vi "State Machine.vi"() -> ()   [LabVIEW 2018]
uses:
  <vilib>/Platform/TimedLoop/XDataNode/timing_clust.ctl
  <vilib>/Platform/TimedLoop/XDataNode/nitl_modes.ctl
  <vilib>/Platform/TimedLoop/XDataNode/wakeup.ctl
  <extravilib>/ChannelInstances/Tag-bool/Write With Abort.vi
  <extravilib>/ChannelInstances/Tag-a[.](dbl)/Read With Abort.vi
  <extravilib>/ChannelInstances/Tag-a[.](dbl)/Write With Abort.vi
  <extravilib>/ChannelInstances/Tag-bool/Read With Abort.vi
  <extravilib>/ChannelInstances/Tag-bool/Instantiate.vi
  <extravilib>/ChannelInstances/Tag-a[.](dbl)/Instantiate.vi
  <extravilib>/ChannelInstances/Tag-bool/EndpointRead.vi
  <extravilib>/ChannelInstances/Tag-a[.](dbl)/EndpointRead.vi
  <extravilib>/ChannelInstances/Tag-bool/Endpoint.vi
  <extravilib>/ChannelInstances/Tag-a[.](dbl)/Endpoint.vi
  <vilib>/Platform/TimedLoop/XDataNode/XDataNode.xnode
  <extravilib>/ChannelInstances/Tag-bool.lvlib
  <vilib>/Platform/TimedLoop/XDataNode/XDNodeRunTimeDep.lvlib
  <extravilib>/ChannelInstances/Tag-a[.](dbl).lvlib
panel:
  in  "Reset Button":bool
  out "State":enum16{"Start", "NE", "SE", "NW", "SW", "Reset"}(ring)
  out "error out":errorcluster
  in  "Stop Button":bool
  out "Calibrated":bool=TRUE
  in  "GO?":bool
  out "Stitched Image":T1(plugin-control)
  out "Acquired Image":T1(plugin-control)
  # "Mechatronic Systems Board"
  # "State Machines"
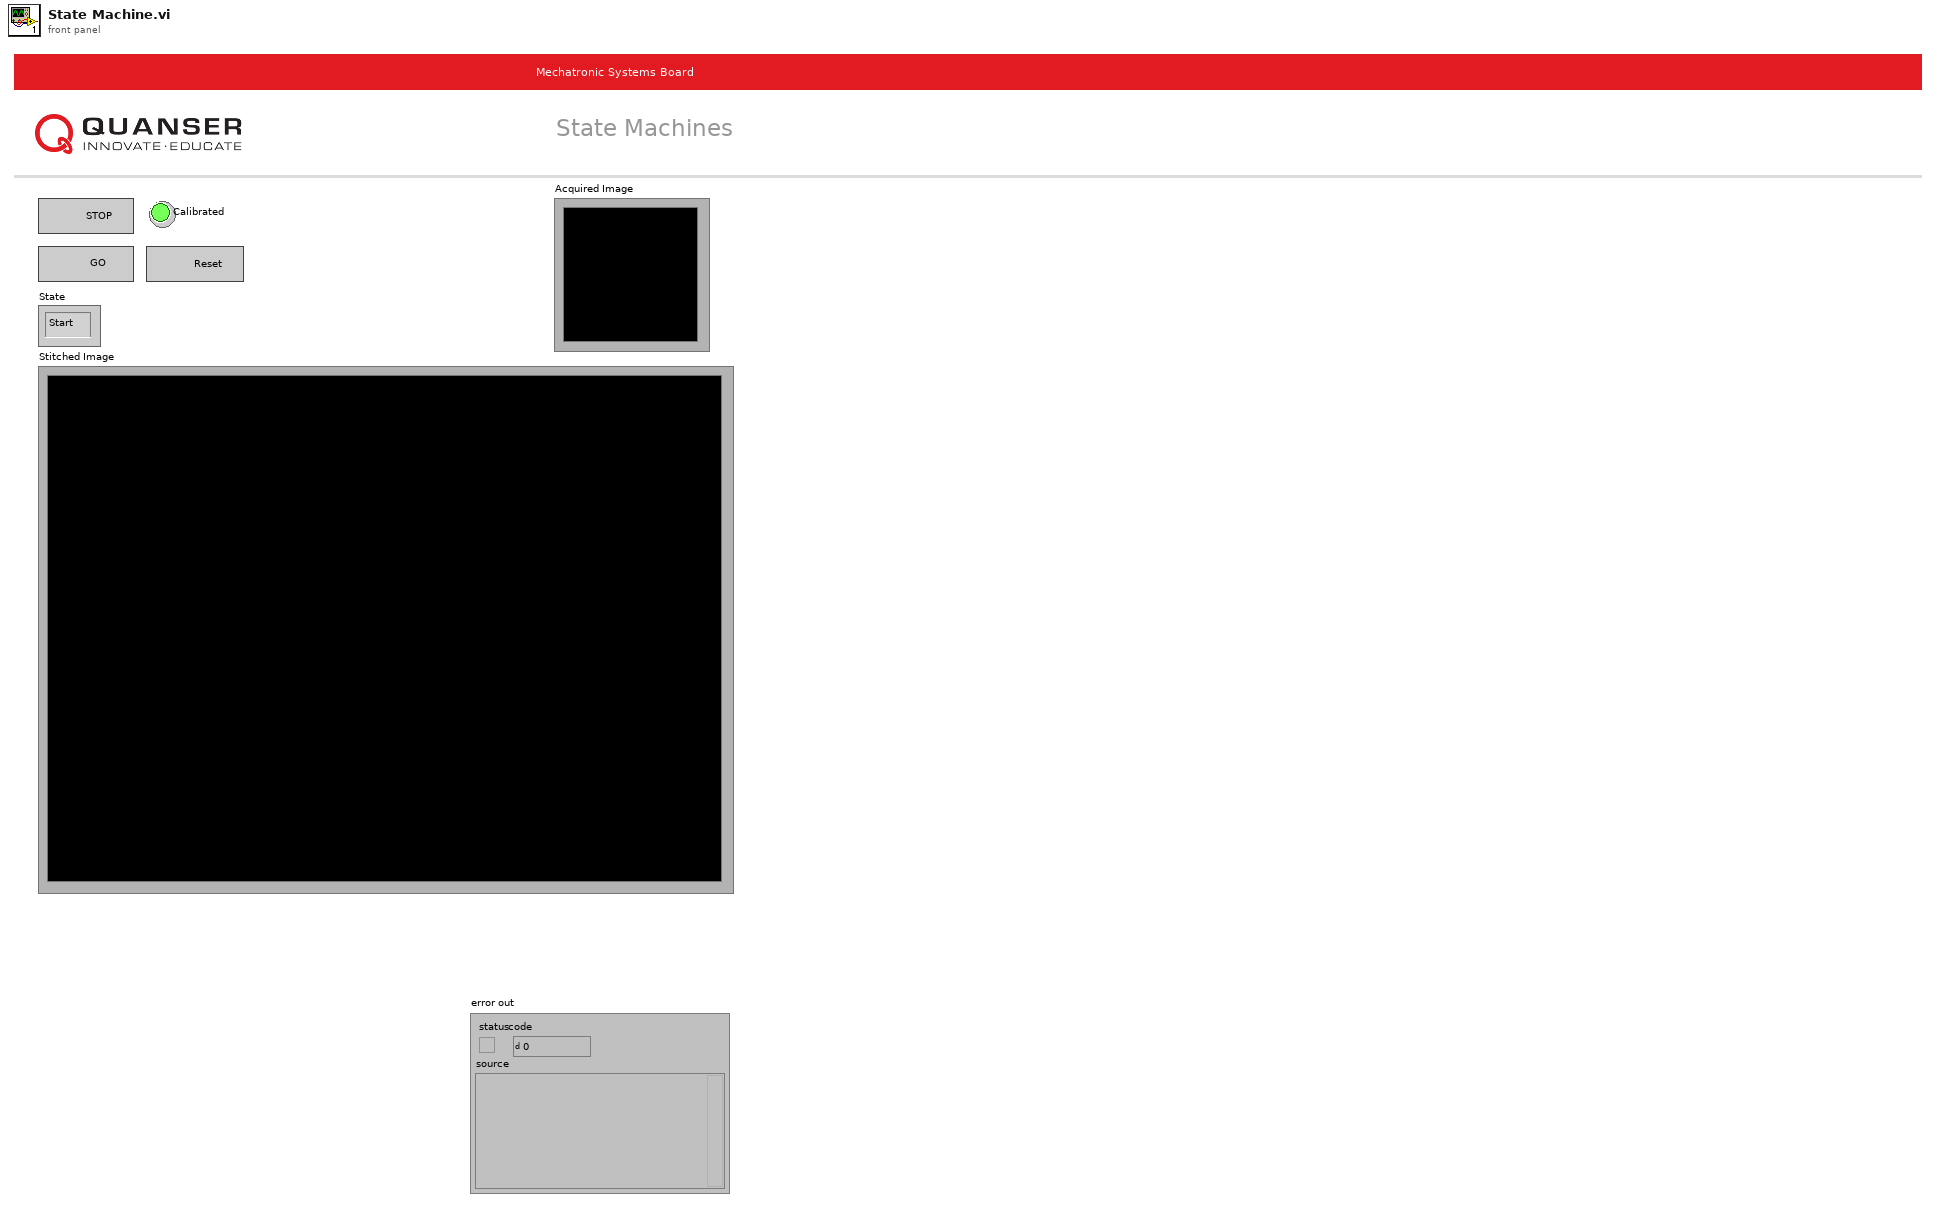
[diagram p1: front panel]
types:
  T1 = typedef "IMAQ Image.ctl" = refnum<image>
  T2 = typedef "QNET MS IO Cluster.ctl" = cluster{"Error":errorcluster, "Encoder Calibration Values":i32[], "Update Calibration":bool, "JPEG Resolutions":u16, "Raw Resolutions":u16, "Image Mode":enum16{"RAW RGB", "RAW Gray Scale", "JPEG"}, "FPGA Ref":refnum<k20>}
  T3 = typedef "XDNodeRunTimeDep.lvlib/timing_clust.ctl" = cluster{"Expected End [f-1]":u64, "Actual End [f-1]":u64, "Finished Late? [f-1]":bool, "Expected End [i-1]":u64, "Actual End [i-1]":u64, "Finished Late? [i-1]":bool, "Expected Start [i]":u64, "Actual Start [i]":u64, "Expected Start [f]":u64, "Actual Start [f]":u64, "Source Name":string, "Structure Name":string, "Period":i64, "Deadline":i64, "Offset":i64, "Start":i64, "Priority":i32, "Timeout":i32, "Mode":T4, "Wakeup Reason":T5, "Error":errorcluster, "Source Type":string, "Secondary Source Type":string, "Global End Time":u64, "Global Start Time":u64, "Frame Duration":u64, "Iteration Duration":u64, "Assigned CPU":i32, "I/O Scan Engine Mode":u32}
  T4 = typedef "XDNodeRunTimeDep.lvlib/nitl_modes.ctl" = enum32{"No Change", "Process missed periods, maintain original phase", "Discard missed periods, maintain original phase", "Process missed periods, ignore original phase", "Discard missed periods, ignore original phase"}
  T5 = typedef "XDNodeRunTimeDep.lvlib/wakeup.ctl" = enum32{"Normal", "Aborted", "Asynchronous wakeup", "Timing source error", "Timed loop error", "Timeout"}
  T6 = typedef "Tag-a[.](dbl).lvlib/))Channel.ctl" = refnum<queue>
  T7 = typedef "Tag-bool.lvlib/))Channel.ctl" = refnum<queue>
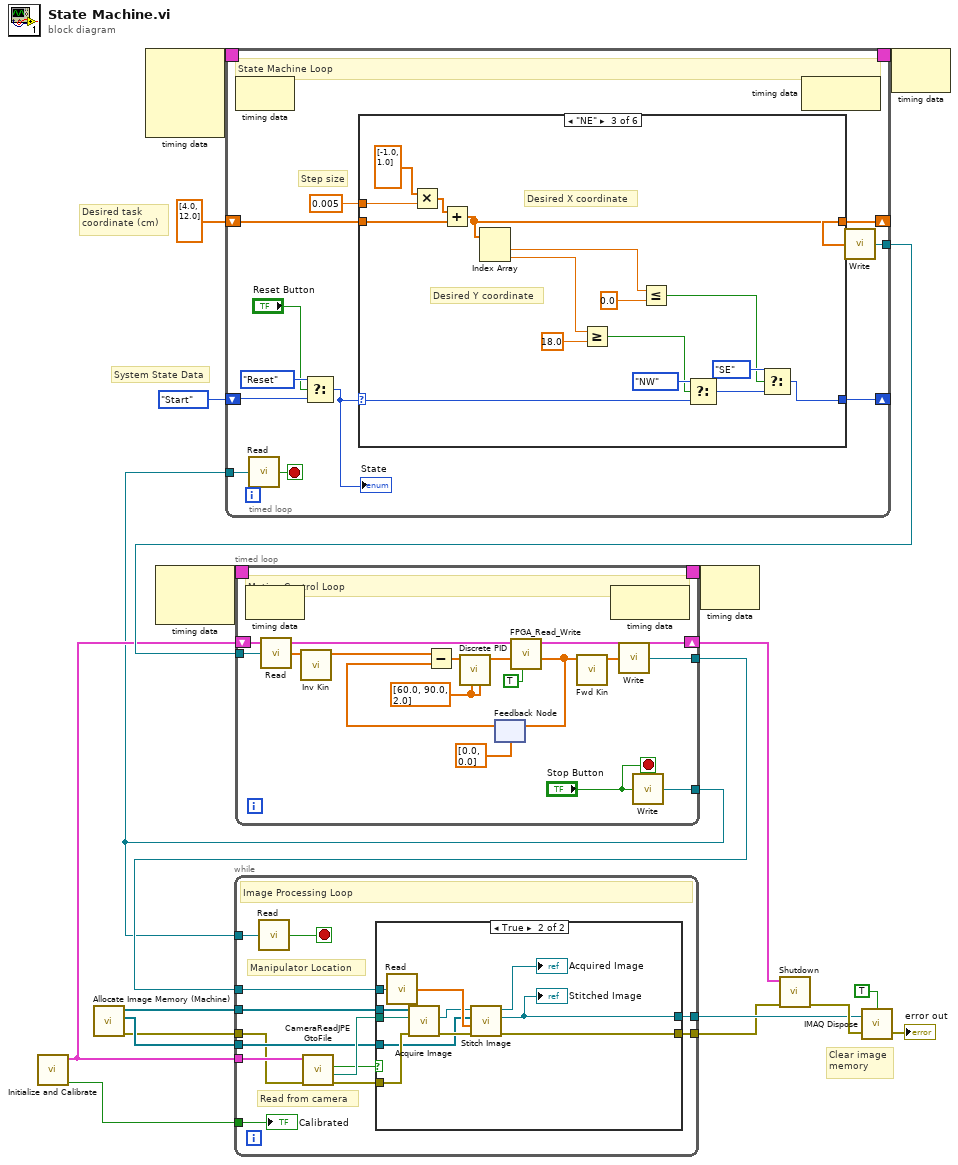
[diagram p0: block diagram]
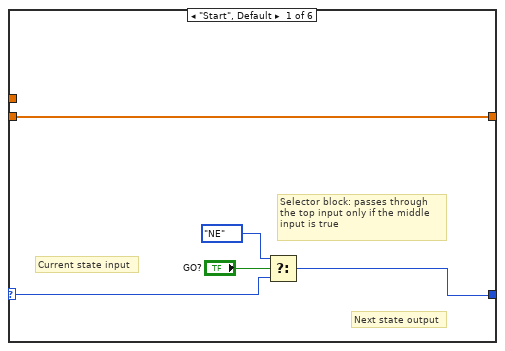
[diagram p2: hidden frame]
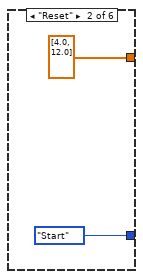
[diagram p3: hidden frame]
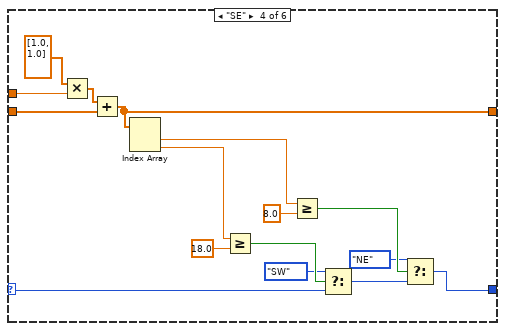
[diagram p4: hidden frame]
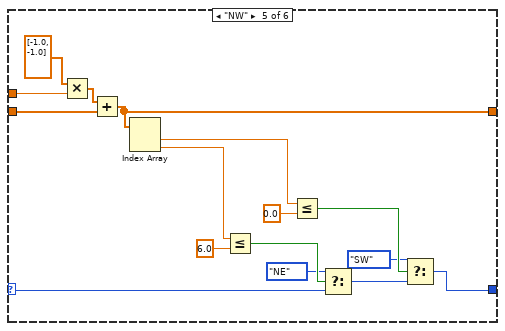
[diagram p5: hidden frame]
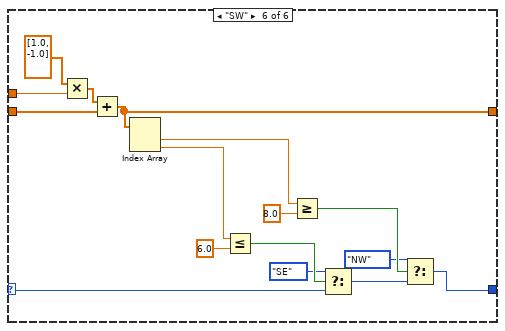
[diagram p6: hidden frame]
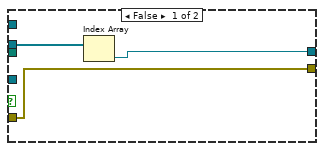
[diagram p7: hidden frame]
diagram:
  # "System State Data"
  # "Desired task \ncoordinate (cm)"
  # "Clear image\nmemory"
  n1 = call "Initialize and Calibrate.vi"() -> ("Calibrated"=w4:bool, "IO Cluster"=w11:T2)  [unwired: 10 in]
  n2 = call "Allocate Image Memory (Machine).vi"() -> ("error out"=w17:errorcluster, "Process Memory"=w18:T1[], "Acquisition Memory"=w19:T1[])  [unwired: 9 in]
  n3 = node-c288() -> (w3:T3)  [unwired: 4 in]
  n4 = node-c288() -> (w16:T3)  [unwired: 2 in]
  n5 = timed-loop {
    tunnel: w9 -> [w31]
    tunnel: [w27] -> w14
    shift-right: [w28] -> _
    shift-left: dbl[] [4.0, 12.0] ("t") -> [w29]
    shift-right: [w25] -> _
    shift-left: enum16{"Start", "NE", "SE", "NW", "SW", "Reset"}."Start" ("t") -> [w23]
    timing: w3 -> [_]
    timing-out: [_] -> w2
    stop <- w30 stop-if-true
    # "Step size"
    # "State Machine Loop"
    n6 = node-c288() -> ()  [unwired: 1 in, 1 out]
    n7 = call <extravilib>:"Read.vi"("channel"=w31) -> ("element"=w30:bool)  [unwired: 1 in, 1 out]
    n8 = Select(t=enum16{"Start", "NE", "SE", "NW", "SW", "Reset"}."Reset", s="Reset Button", f=w23) -> (s? t:f=w24:enum16{"Start", "NE", "SE", "NW", "SW", "Reset"})
    "State" <- w24
    n9 = case shown="\"NE\"" w24 {
      selector: w24 -> [w35 _ w55 w67 w83 w99]
      tunnel: w29 -> [w38 _ w47 w58 w74 w90]
      tunnel: [w38 dbl[] [4.0, 12.0] ("t") w46 w57 w73 w89] -> w28
      tunnel: [w34 enum16{"Start", "NE", "SE", "NW", "SW", "Reset"}."Start" ("t") w53 w64 w80 w96] -> w25
      tunnel: 0.005 ("y") -> [_ _ w50 w61 w77 w93]
      frame "Start", Default {
        # "Next state output"
        # "Current state input"
        # "Selector block: passes through\nthe top input only if the middle\ninput is true"
        n10 = Select(t=enum16{"Start", "NE", "SE", "NW", "SW", "Reset"}."NE", s="GO?", f=w35) -> (s? t:f=w34:enum16{"Start", "NE", "SE", "NW", "SW", "Reset"})
      }
      frame "Reset" {
      }
      frame "NE" {
        # "Desired Y coordinate"
        # "Desired X coordinate"
        n11 = Multiply(x=dbl[] [-1.0, 1.0], y=w50) -> (x*y=w52:dbl[])
        n12 = Add(x=w52, y=w47) -> (x+y=w46:dbl[])
        n13 = Index Array(array=w46) -> (element #1=w44:dbl, element #2=w41:dbl)  [unwired: 2 in]
        n14 = Greater Or Equal?(x=w41, y=18.0) -> (x >= y?=w43:bool)
        n15 = Less Or Equal?(x=w44, y=0.0) -> (x <= y?=w42:bool)
        n16 = Select(t=enum16{"Start", "NE", "SE", "NW", "SW", "Reset"}."NW", s=w43, f=w55) -> (s? t:f=w54:enum16{"Start", "NE", "SE", "NW", "SW", "Reset"})
        n17 = Select(t=enum16{"Start", "NE", "SE", "NW", "SW", "Reset"}."SE", s=w42, f=w54) -> (s? t:f=w53:enum16{"Start", "NE", "SE", "NW", "SW", "Reset"})
      }
      frame "SE" {
        n18 = Multiply(x=dbl[] [1.0, 1.0], y=w61) -> (x*y=w63:dbl[])
        n19 = Add(x=w63, y=w58) -> (x+y=w57:dbl[])
        n20 = Index Array(array=w57) -> (element #1=w72:dbl, element #2=w71:dbl)  [unwired: 2 in]
        n21 = Greater Or Equal?(x=w71, y=18.0) -> (x >= y?=w68:bool)
        n22 = Greater Or Equal?(x=w72, y=8.0) -> (x >= y?=w66:bool)
        n23 = Select(t=enum16{"Start", "NE", "SE", "NW", "SW", "Reset"}."SW", s=w68, f=w67) -> (s? t:f=w65:enum16{"Start", "NE", "SE", "NW", "SW", "Reset"})
        n24 = Select(t=enum16{"Start", "NE", "SE", "NW", "SW", "Reset"}."NE", s=w66, f=w65) -> (s? t:f=w64:enum16{"Start", "NE", "SE", "NW", "SW", "Reset"})
      }
      frame "NW" {
        n25 = Multiply(x=dbl[] [-1.0, -1.0], y=w77) -> (x*y=w79:dbl[])
        n26 = Add(x=w79, y=w74) -> (x+y=w73:dbl[])
        n27 = Index Array(array=w73) -> (element #1=w88:dbl, element #2=w87:dbl)  [unwired: 2 in]
        n28 = Less Or Equal?(x=w87, y=6.0) -> (x <= y?=w84:bool)
        n29 = Less Or Equal?(x=w88, y=0.0) -> (x <= y?=w82:bool)
        n30 = Select(t=enum16{"Start", "NE", "SE", "NW", "SW", "Reset"}."NE", s=w84, f=w83) -> (s? t:f=w81:enum16{"Start", "NE", "SE", "NW", "SW", "Reset"})
        n31 = Select(t=enum16{"Start", "NE", "SE", "NW", "SW", "Reset"}."SW", s=w82, f=w81) -> (s? t:f=w80:enum16{"Start", "NE", "SE", "NW", "SW", "Reset"})
      }
      frame "SW" {
        n32 = Multiply(x=dbl[] [1.0, -1.0], y=w93) -> (x*y=w95:dbl[])
        n33 = Add(x=w95, y=w90) -> (x+y=w89:dbl[])
        n34 = Index Array(array=w89) -> (element #1=w104:dbl, element #2=w103:dbl)  [unwired: 2 in]
        n35 = Less Or Equal?(x=w103, y=6.0) -> (x <= y?=w100:bool)
        n36 = Greater Or Equal?(x=w104, y=8.0) -> (x >= y?=w98:bool)
        n37 = Select(t=enum16{"Start", "NE", "SE", "NW", "SW", "Reset"}."SE", s=w100, f=w99) -> (s? t:f=w97:enum16{"Start", "NE", "SE", "NW", "SW", "Reset"})
        n38 = Select(t=enum16{"Start", "NE", "SE", "NW", "SW", "Reset"}."NW", s=w98, f=w97) -> (s? t:f=w96:enum16{"Start", "NE", "SE", "NW", "SW", "Reset"})
      }
    }
    n39 = node-c288() -> ()  [unwired: 1 in, 1 out]
    n40 = call <extravilib>:"Write.vi"("element"=w28) -> ("channel"=w27:T6)  [unwired: 1 out]
  }
  n41 = timed-loop {
    timing: w16 -> [_]
    timing-out: [_] -> w15
    tunnel: [w111] -> w13
    tunnel: w14 -> [w110]
    shift-right: [w116] -> w12
    shift-left: w11 -> [w108]
    tunnel: [w106] -> w9
    stop <- "Stop Button" stop-if-true
    w105 = dbl[] [60.0, 90.0, 2.0] ("Gains Motor 0")
    # "Motion Control Loop"
    n42 = node-c288() -> ()  [unwired: 1 in, 1 out]
    n43 = call <extravilib>:"Read.vi"("channel"=w110) -> ("element"=w109:dbl[])  [unwired: 1 in, 1 out]
    n44 = call "Inv Kin.vi"("Task Coordinates (cm)"=w109) -> ("Joint Coordinates (rad)"=w117:dbl[])  [unwired: 10 in]
    n45 = feedback #1(dbl[] [0.0, 0.0] ("Joint Coordinates (rad)")) -> (w115:dbl[])
    n46 = Subtract(x=w117, y=w115) -> (x-y=w118:dbl[])
    n47 = call "Discrete PID.vi"("Gains Motor 1"=w105, "Gains Motor 0"=w105, "Error Array"=w118) -> ("Voltage"=w119:dbl[])  [unwired: 8 in]
    n48 = call "FPGA_Read_Write.vi"("Motors enabled?"=TRUE, "Commands"=w119, "IO Cluster In"=w108) -> ("Joint Coordinates (rad)"=w114:dbl[], "IO Cluster Out"=w116:T2)  [unwired: 5 in, 2 out]
    n49 = feedback-in #1(w114) -> ()
    n50 = call "Fwd Kin.vi"("Joint Coordinates (rad)"=w114) -> ("Task Coordinates (cm)"=w112:dbl[])  [unwired: 9 in, 1 out]
    n51 = node-c288() -> ()  [unwired: 1 in, 1 out]
    n52 = call <extravilib>:"Write.vi"("element"=w112) -> ("channel"=w111:T6)  [unwired: 1 out]
    n53 = call <extravilib>:"Write.vi"("element"="Stop Button") -> ("channel"=w106:T7)  [unwired: 1 out]
  }
  n54 = while {
    tunnel: w11 -> [w135]
    tunnel: [w131] -> w6
    tunnel: w19 -> [w130]
    tunnel: w18 -> [w129]
    tunnel: w17 -> [w128]
    tunnel: w13 -> [w127]
    tunnel: w9 -> [w126]
    tunnel: [w124] -> w7
    tunnel: w4 -> [w123]
    stop <- w125 stop-if-true
    # "Read from camera"
    # "Manipulator Location"
    # "Image Processing Loop"
    n55 = call <extravilib>:"Read.vi"("channel"=w126) -> ("element"=w125:bool)  [unwired: 1 in, 1 out]
    n56 = call "CameraReadJPEGtoFile.vi"("error in"=w128, "IO Cluster In"=w135) -> ("Error Out"=w132:errorcluster, "Image File"=w134:path, "New Image Data"=w133:bool)  [unwired: 6 in, 1 out]
    n57 = case shown="True" w133 {
      tunnel: w134 -> [_ w148]
      tunnel: w132 -> [w136 w149]
      tunnel: [w136 w141] -> w131
      tunnel: w130 -> [w138 w147]
      tunnel: w129 -> [_ w140]
      tunnel: w127 -> [_ w146]
      tunnel: [w137 w142] -> w124
      frame False {
        n58 = Index Array(array=w138) -> (element=w137:T1)  [unwired: 1 in]
      }
      frame True {
        n59 = call <extravilib>:"Read.vi"("channel"=w146) -> ("element"=w144:dbl[])  [unwired: 1 in, 1 out]
        n60 = call "Acquire Image.vi"("Error In"=w149, "File Path"=w148, "Acquisition Memory"=w147) -> ("Error Out"=w145:errorcluster, "HSL Image"=w139:T1)  [unwired: 4 in, 3 out]
        n61 = call "Stitch Image.vi"("Error In"=w145, "Manipulator Location"=w144, "Process Memory"=w140, "Source Image"=w139) -> ("Error Out"=w141:errorcluster, "Stitched Image"=w142:T1, "Acquired Image"=→"Acquired Image":T1)  [unwired: 5 in]
        "Stitched Image" <- w142
      }
    }
    "Calibrated" <- w123
  }
  n62 = node-c288(w15) -> ()  [unwired: 1 out]
  n63 = call "Shutdown.vi"("Image Processing Loop"=w6, "IO Cluster In"=w12) -> ("Error"=w10:errorcluster)  [unwired: 9 in]
  n64 = call "IMAQ Dispose"("All Images? (No)"=TRUE, "Image"=w7, "error in (no error)"=w10) -> ("error out"=→"error out":errorcluster)  [unwired: 3 in]
  n65 = node-c288(w2) -> ()  [unwired: 1 out]
